vi "2D Gaussian - Fit Image U16.vi"(7 "Image In (U16)":u16[][](array[numeric]), 11 "Error In":errorcluster) -> (8 "Best Fit Params":T1, 15 "Error Out":errorcluster)   [LabVIEW 2016]
uses:
  2D Gaussian - Type Defs/2D Gaussian - Best Fit Parameters.ctl
  <vilib>/gmath/NumericalOptimization/Nonlinear Curve Fit LM bound.vi
  <vilib>/gmath/NI_Gmath.lvlib
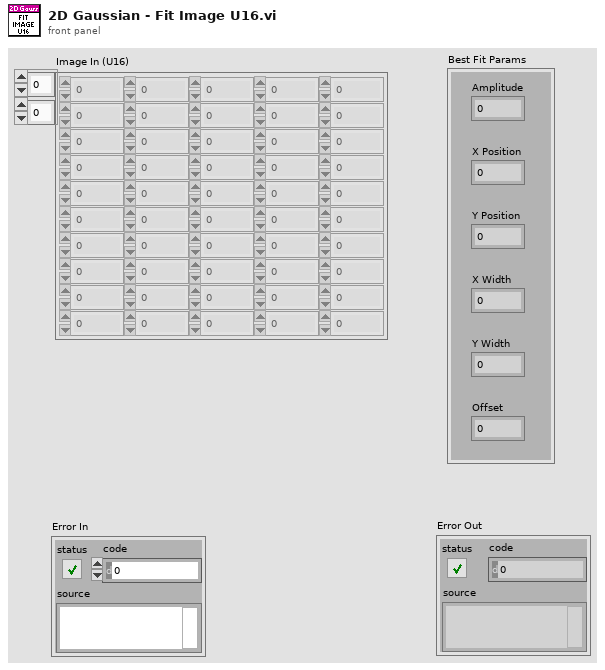
[diagram p1: front panel]
types:
  T1 = typedef "2D Gaussian - Best Fit Parameters.ctl" = cluster{"Amplitude":dbl, "X Position":dbl, "Y Position":dbl, "X Width":dbl, "Y Width":dbl, "Offset":dbl}
  T2 = cluster{"parameter minimum":dbl[], "parameter maximum":dbl[]}
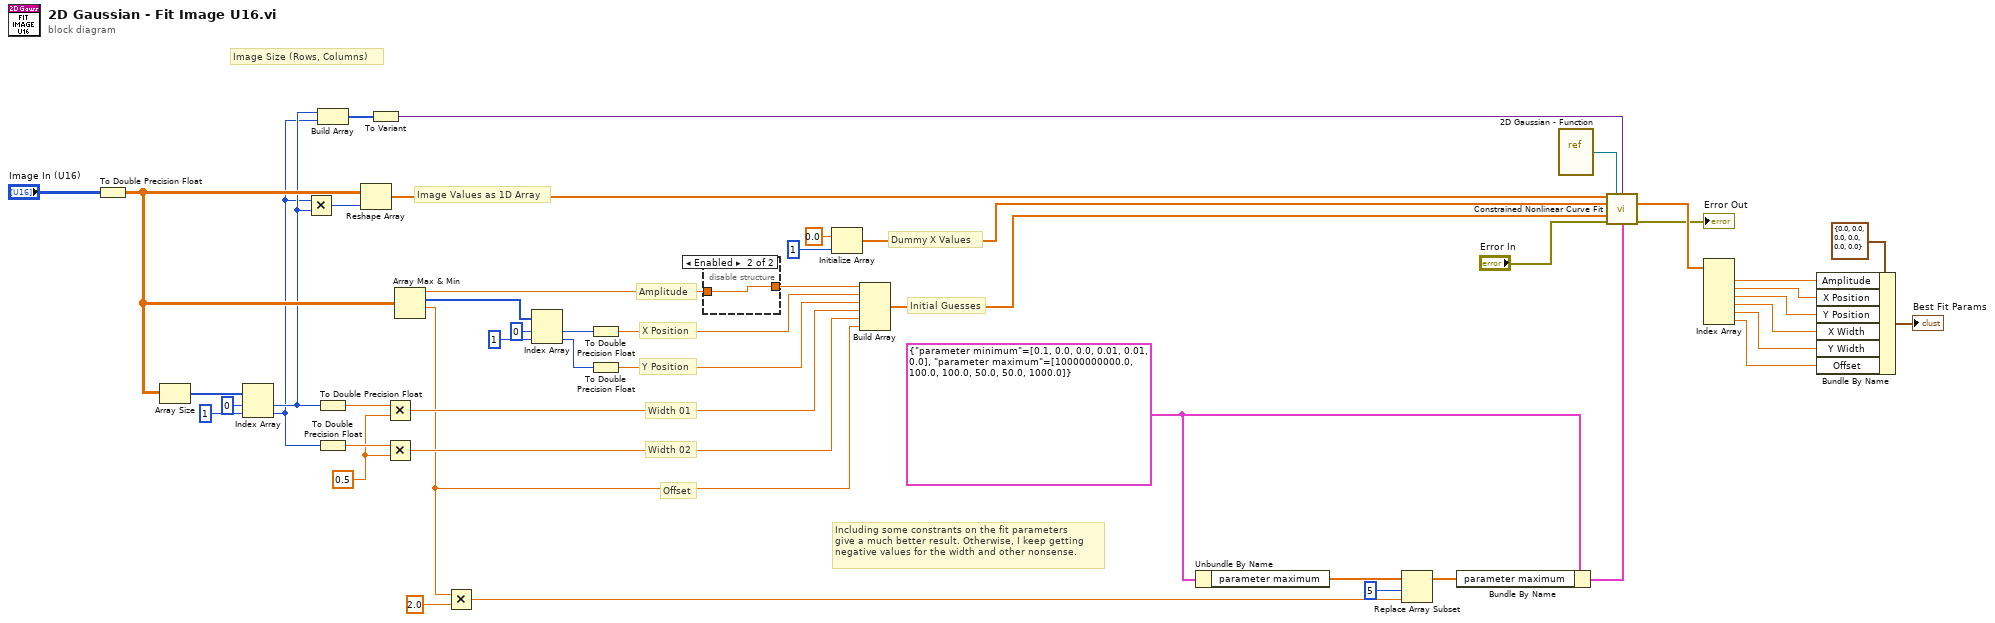
[diagram p0: block diagram]
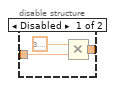
[diagram p2: hidden frame]
diagram:
  w8 = T2 {"parameter minimum"=[0.1, 0.0, 0.0, 0.01, 0.01, 0.0], "parameter maximum"=[10000000000.0, 100.0, 100.0, 50.0, 50.0, 1000.0]} ("parameter bounds")
  w33 = 0.5
  # "Image Size (Rows, Columns)"
  # "Including some constrants on the fit parameters\ngive a much better result. Otherwise, I keep getting\nnegative values for the width and other nonsense."
  # "Dummy X Values"
  # "Image Values as 1D Array"
  # "Initial Guesses"
  # "Width 02"
  # "Width 01"
  # "Y Position"
  # "X Position"
  # "Offset"
  # "Amplitude"
  n1 = To Double Precision Float(number="Image In (U16)") -> (double precision float=w26:dbl[][])
  n2 = Array Size(array=w26) -> (size(s)=w36:i32[])
  n3 = Index Array(array=w36, index #1=0 ("index"), index #2=1 ("index")) -> (element #1=w24:i32, element #2=w23:i32)
  n4 = Multiply(x=w23, y=w24) -> (x*y=w29:i32)
  n5 = Build Array(w24, w23) -> (w22:i32[])
  n6 = To Double Precision Float(number=w24) -> (double precision float=w35:dbl)
  n7 = To Double Precision Float(number=w23) -> (double precision float=w34:dbl)
  n8 = Reshape Array(w26, w29) -> (w30:dbl[])
  n9 = To Variant(anything=w22) -> (Variant=w21:variant)
  n10 = Multiply(x=w35, y=w33) -> (x*y=w32:dbl)
  n11 = Multiply(x=w34, y=w33) -> (x*y=w31:dbl)
  n12 = Array Max & Min(array=w26) -> (max value=w47:dbl, max index (indices)=w45:i32[], min value=w10:dbl)  [unwired: 1 out]
  n13 = Multiply(x=w10, y=2.0) -> (x*y=w4:dbl)
  n14 = Index Array(array=w45, index #1=0 ("index"), index #2=1 ("index")) -> (element #1=w42:i32, element #2=w40:i32)
  n15 = To Double Precision Float(number=w42) -> (double precision float=w41:dbl)
  n16 = To Double Precision Float(number=w40) -> (double precision float=w39:dbl)
  n17 = disable-structure shown="Enabled" {
    disable-tunnel: w47 -> [w51 w53]
    disable-tunnel: [w50 w53] -> w46
    frame Disabled {
      n18 = Multiply(x=3.141592653589793, y=w51) -> (x*y=w50:dbl)
    }
    frame Enabled {
    }
  }
  n19 = Initialize Array(0.0 ("element"), 1 ("dimension size")) -> (w27:dbl[])
  n20 = Build Array(w46, w41, w39, w32, w31, w10) -> (w25:dbl[])
  n21 = Unbundle By Name(w8) -> ("parameter maximum"=w7:dbl[])
  n22 = Replace Array Subset(array=w7, new element=w4, index=5) -> (w6:dbl[])
  n23 = Bundle By Name(cluster=w8, "parameter maximum"=w6) -> (w3:T2)
  n24 = vi-ref "2D Gaussian - Function.vi"() -> (w49:refnum<vi>)
  n25 = call-poly <vilib>:"Constrained Nonlinear Curve Fit.vi"("Y"=w30, "f(x,a)"=w49, "data"=w21, "X"=w27, "initial parameters"=w25, "error in (no error)"="Error In", "parameter bounds"=w3) -> ("best fit parameters"=w19:dbl[], "error out"=→"Error Out":errorcluster)  [unwired: 3 in, 4 out]
  n26 = Index Array(array=w19) -> (element #1=w18:dbl, element #2=w17:dbl, element #3=w16:dbl, element #4=w15:dbl, element #5=w14:dbl, element #6=w13:dbl)  [unwired: 6 in]
  n27 = Bundle By Name(cluster=T1 {"Amplitude"=0.0, "X Position"=0.0, "Y Position"=0.0, "X Width"=0.0, "Y Width"=0.0, "Offset"=0.0} ("Best Fit Parameters"), "Amplitude"=w18, "X Position"=w17, "Y Position"=w16, "X Width"=w15, "Y Width"=w14, "Offset"=w13) -> (→"Best Fit Params":T1)
